vi "livevideo.vi"(0 "stop":bool, 1 "Camera ID":u32=285941632) -> (2 "image out":picture)   [LabVIEW 2015]
uses:
  <vilib>/picture/picture.llb/imagedata.ctl
  <vilib>/Utility/miscctls.llb/LVPointTypeDef.ctl
panel:
  in  "Snapshot":bool
  in  "Zoom":sgl(slide)=33.0 min=0 step=1 scale=0.0..300.0
  in  "Fit":bool
  in  "Video Mode":i32(listbox)=35
  in  "image data":T1={"image type"=0, "image depth"=24, "image"=[], "mask"=[], "colors"=[], "Rectangle"={"left"=0, "top"=0, "right"=0, "bottom"=0}}
  out "Loading":string
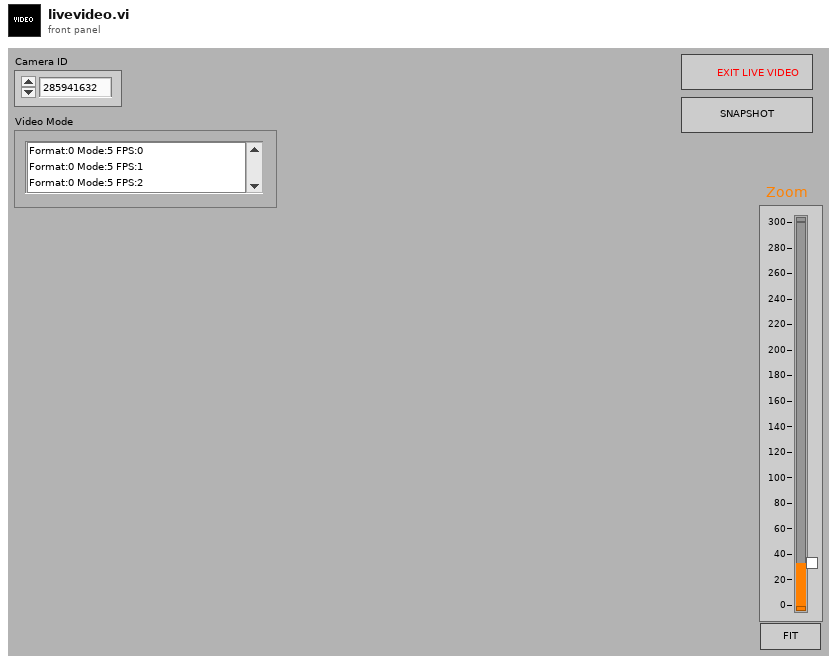
[diagram p1: front panel]
types:
  T1 = typedef "imagedata.ctl" = cluster{"image type":i32, "image depth":i32, "image":u8[], "mask":u8[], "colors":u32[], "Rectangle":cluster{"left":i16, "top":i16, "right":i16, "bottom":i16}}
  T2 = typedef "LVPointTypeDef.ctl" = cluster{"Horizontal":i16, "Vertical":i16}
  T3 = cluster{"left":i16, "top":i16, "right":i16, "bottom":i16}
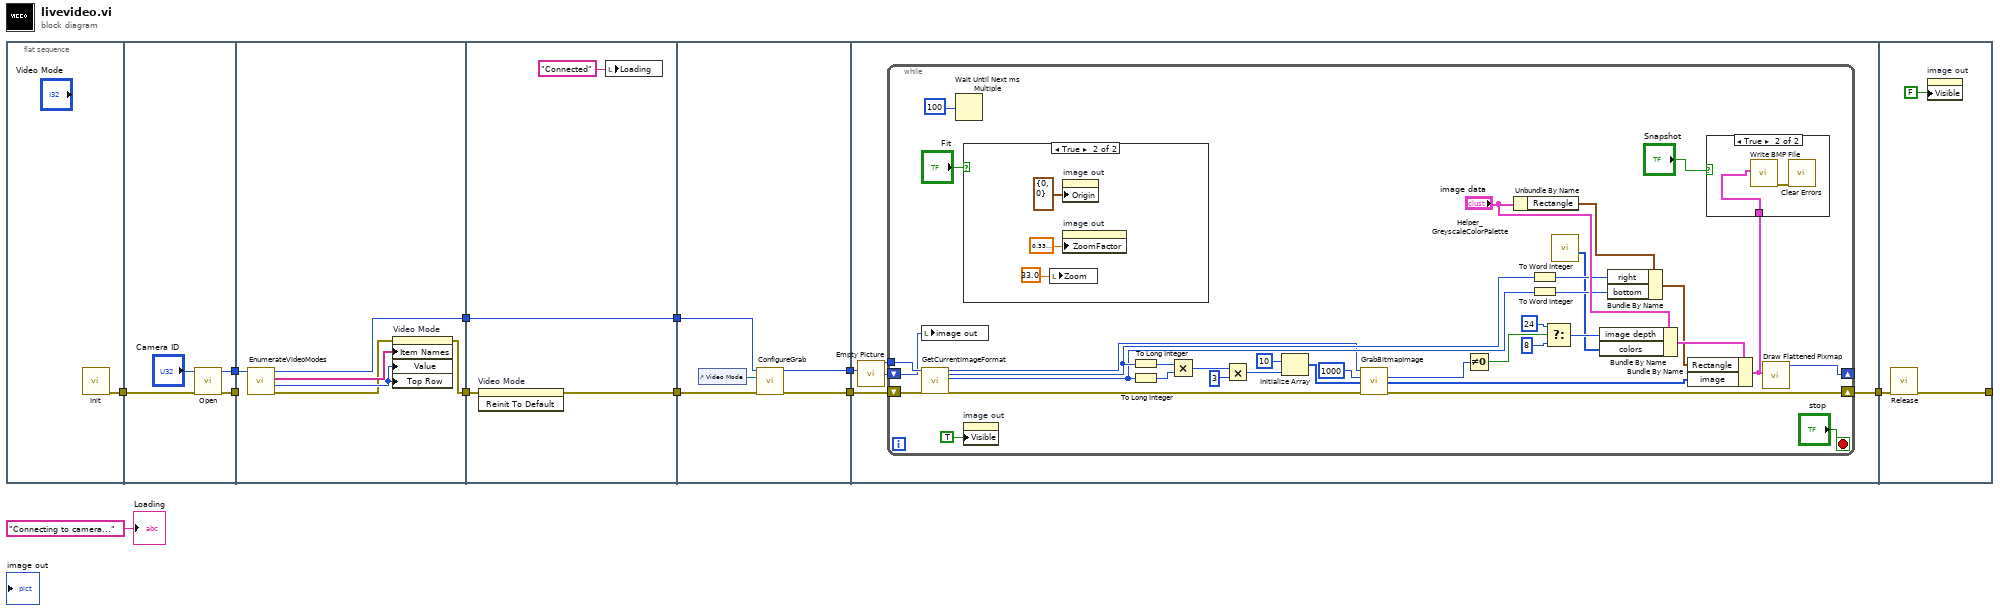
[diagram p0: block diagram]
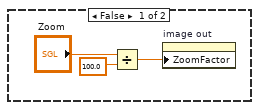
[diagram p3: hidden frame]
diagram:
  n1 = flat-sequence {
    tunnel: [w12] -> w11
    tunnel: w11 -> [w14]
    tunnel: [w16] -> w10
    tunnel: [w13] -> w9
    tunnel: w10 -> [_]
    tunnel: w9 -> [w20]
    tunnel: [w19] -> w6
    tunnel: [w17] -> w5
    tunnel: [w26] -> w4
    tunnel: [w23] -> w3
    tunnel: w5 -> [w24]
    tunnel: w6 -> [w26]
    tunnel: [w28] -> w8
    tunnel: [w30] -> w7
    tunnel: w4 -> [w31]
    tunnel: w3 -> [w29]
    tunnel: w8 -> [w34]
    tunnel: w7 -> [w35]
    tunnel: [w33] -> w2
    tunnel: [w82] -> _
    tunnel: w2 -> [w81]
    frame #0 {
      n2 = call <userlib>:"Init.vi"() -> ("error out"=w12:errorcluster)  [unwired: 11 out]
    }
    frame #1 {
      n3 = call <userlib>:"Open.vi"("error in (no error)"=w14, "CamId"="Camera ID") -> ("error out"=w16:errorcluster, "CamId out"=w13:u32)  [unwired: 1 in, 7 out]
    }
    frame #2 {
      n4 = call <userlib>:"EnumerateVideoModes.vi"("CamId"=w20) -> ("error out"=w18:errorcluster, "Current Mode"=w22:i32, "Video Modes"=w21:string[], "CamId out"=w19:u32)  [unwired: 2 in, 5 out]
      n5 = property on="Video Mode" class="LstBox (strict)"(error in=w18, "Item Names"=w21, "Value"=w22, "Top Row"=w22) -> (error out=w17:errorcluster)  [unwired: 1 in, 1 out]
    }
    frame #3 {
      n6 = invoke on="Video Mode" class="LstBox (strict)" method="Reinit To Default"(error in=w24) -> (error out=w23:errorcluster)  [unwired: 2 in, 2 out]
      n7 = local write "Loading"("Connected" ("Loading")) -> ()
    }
    frame #4 {
      n8 = control-ref of="Video Mode"() -> (w27:refnum<vi>)
      n9 = call <userlib>:"ConfigureGrab.vi"("CamId"=w31, "Video Modes"=w27, "error in (no error)"=w29) -> ("CamId out"=w30:u32, "error out"=w28:errorcluster)  [unwired: 11 out]
    }
    frame #5 {
      n10 = call "Empty Picture"() -> ("empty picture"=w32:picture)
      n11 = while {
        tunnel: w35 -> [w61]
        shift-right: [w45] -> w33
        shift-left: w34 -> [w44]
        shift-right: [w40] -> _
        shift-left: w32 -> [w41]
        stop <- "stop" stop-if-true
        n12 = local write "image out"(w41) -> ()
        n13 = call <userlib>:"GetCurrentImageFormat.vi"("CamId"=w61, "error in (no error)"=w44) -> ("CamId out"=w48:u32, "pnImageWidth"=w71:u32, "pnImageHeight"=w70:u32, "error out"=w46:errorcluster)  [unwired: 14 out]
        n14 = Wait Until Next ms Multiple(millisecond multiple=u32 100) -> ()  [unwired: 1 out]
        n15 = case shown="True" "Fit" {
          frame False {
            n16 = Divide(x="Zoom", y=sgl 100.0) -> (x/y=w74:sgl)
            n17 = property on="image out" class="Pict"("ZoomFactor"=w74) -> ()  [unwired: 2 in, 2 out]
          }
          frame True {
            n18 = local write "Zoom"(sgl 33.0 ("Zoom")) -> ()
            n19 = property on="image out" class="Pict"("Origin"=T2 {"Horizontal"=0, "Vertical"=0}) -> ()  [unwired: 2 in, 2 out]
            n20 = property on="image out" class="Pict"("ZoomFactor"=sgl 0.33 ("Zoom Factor")) -> ()  [unwired: 2 in, 2 out]
          }
        }
        n21 = property on="image out" class="Pict"("Visible"=TRUE) -> ()  [unwired: 2 in, 2 out]
        n22 = To Long Integer(number=w71) -> (32bit integer=w65:i32)
        n23 = To Long Integer(number=w70) -> (32bit integer=w66:i32)
        n24 = Multiply(x=w65, y=w66) -> (x*y=w68:i32)
        n25 = Multiply(x=w68, y=3) -> (x*y=w64:i32)
        n26 = Initialize Array(u8 10 ("element"), w64) -> (w63:u8[])
        n27 = call <userlib>:"GrabBitmapImage.vi"("CamId"=w48, "nTimeOut"=u32 1000, "pImage In"=w63, "error in (no error)"=w46) -> ("pbIsColor"=w53:u32, "pImage"=w52:u8[], "error out"=w45:errorcluster)  [unwired: 1 in, 8 out]
        n28 = Not Equal To 0?(x=w53) -> (x != 0?=w54:bool)
        n29 = Unbundle By Name("image data") -> ("Rectangle"=w59:T3)
        n30 = To Word Integer(number=w71) -> (16bit integer=w50:i16)
        n31 = To Word Integer(number=w70) -> (16bit integer=w49:i16)
        n32 = Select(t=24, s=w54, f=8) -> (s? t:f=w55:i32)
        n33 = call <userlib>:"Helper_GreyscaleColorPalette.vi"() -> ("GreyscaleColorPalette"=w47:u32[])  [unwired: 11 out]
        n34 = Bundle By Name(cluster="image data", "image depth"=w55, "colors"=w47) -> (w58:T1)
        n35 = Bundle By Name(cluster=w59, "right"=w50, "bottom"=w49) -> (w51:T3)
        n36 = Bundle By Name(cluster=w58, "Rectangle"=w51, "image"=w52) -> (w36:T1)
        n37 = case shown="True" "Snapshot" {
          tunnel: w36 -> [_ w73]
          frame False {
          }
          frame True {
            n38 = call <vilib>:"Write BMP File.vi"("image data"=w73) -> ("error out"=w72:errorcluster)  [unwired: 9 in, 1 out]
            n39 = call <vilib>:"Clear Errors.vi"("error in (no error)"=w72) -> ()  [unwired: 5 in, 2 out]
          }
        }
        n40 = call <vilib>:"Draw Flattened Pixmap.vi"("image data"=w36) -> ("new picture"=w40:picture)  [unwired: 1 in, 7 out]
      }
    }
    frame #6 {
      n41 = call <userlib>:"Release.vi"("error in (no error)"=w81) -> ("error out"=w82:errorcluster)  [unwired: 10 out]
      n42 = property on="image out" class="Pict"("Visible"=FALSE) -> ()  [unwired: 2 in, 2 out]
    }
  }
  "Loading" <- "Connecting to camera..." ("Loading")
